vi "Close SysCfg Device.vi"(8 "error in":errorcluster, 11 "Controller in":refnum<class "Controller.lvclass">) -> (0 "error out":errorcluster)   [LabVIEW 2016, in "SMI.lvlib" / "SysCfg Device.lvclass"]
uses:
  SysCfg Device.lvclass
  Controller/Controller.lvclass
  C:/GitHub/SystemManagementAndInformation/source/classes/SysCfg Device/SysCfg Device.lvclass
  SysCfg Device.lvclass/SysCfg Device.ctl
  <vilib>/nisyscfg/Close (System).vi
  <vilib>/nisyscfg/Close (Hardware).vi
  <vilib>/nisyscfg/nisyscfg.lvlib
panel:
  out "Controller out":refnum<class "Controller.lvclass">
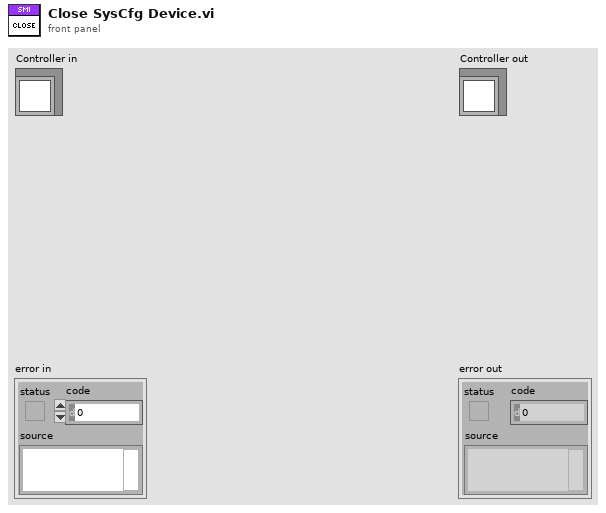
[diagram p1: front panel]
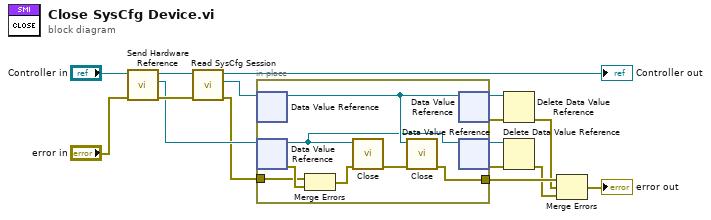
[diagram p0: block diagram]
diagram:
  n1 = call "Send Hardware Reference.vi"("error in"="error in", "Controller in"="Controller in") -> ("error out"=w13:errorcluster, "System Hardware Reference"=w10:refnum<data-value>, "Controller out"=w15:refnum<class "Controller.lvclass">)  [unwired: 7 in]
  n2 = call "Read SysCfg Session.vi"("error in"=w13, "SysCfg Device in"=w15) -> ("error out"=w9:errorcluster, "SysCfg Session"=w11:refnum<data-value>, "SysCfg Device out"=→"Controller out":refnum<class "Controller.lvclass">)  [unwired: 7 in]
  n3 = in-place {
    in-place-border: w9 -> [w22]
    in-place-border: [w19] -> w8
    n4 = in-place-dvr #1(w11) -> (w18:refnum<k21>)  [unwired: 1 out]
    n5 = in-place-dvr #2(w10) -> (w17:refnum<k20>, w23:errorcluster)
    n6 = Merge Errors(w22, w23) -> (w21:errorcluster)
    n7 = call-poly <vilib>:"Close.vi"("error in (no error)"=w21, "Resource in"=w17) -> ("error out"=w20:errorcluster)  [unwired: 9 in]
    n8 = call-poly <vilib>:"Close.vi"("error in (no error)"=w20, "Session in"=w18) -> ("error out"=w19:errorcluster)  [unwired: 9 in]
    n9 = in-place-dvr #1(w18) -> (w6:refnum<data-value>, w5:errorcluster)
    n10 = in-place-dvr #2(w17) -> (w4:refnum<data-value>, w3:errorcluster)
  }
  n11 = Delete Data Value Reference(data value reference=w6, error in=w5) -> (error out=w2:errorcluster)  [unwired: 1 out]
  n12 = Delete Data Value Reference(data value reference=w4, error in=w3) -> (error out=w1:errorcluster)  [unwired: 1 out]
  n13 = Merge Errors(w8, w2, w1) -> (→"error out":errorcluster)
